vi "Get Table Object.vi"(8 "error in (no error)":errorcluster, 11 "Form Model in":refnum<class "Form Model.lvclass">) -> (0 "error out":errorcluster, 2 "Table":refnum<class "Basic Table.lvclass">, 3 "Form Model out":refnum<class "Form Model.lvclass">)   [LabVIEW 2020, in "Form Model.lvlib" / "Form Model.lvclass"]
uses:
  Form Model.lvclass
  Database OOP/Table Libraries/Basic Table/Basic Table Class/Basic Table.lvclass
  Form Model.lvclass/Form Model.ctl
  <vilib>/ActorFramework/Reply Msg/Reply Msg.lvclass/Reply Msg.ctl
  <vilib>/ActorFramework/Message Enqueuer/Message Enqueuer.lvclass/Message Enqueuer.ctl
  <vilib>/ActorFramework/Reply Msg/Send Message And Wait For Response.vi
  <vilib>/ActorFramework/Message Enqueuer/Enqueue.vi
  Panel Form Controller Messages/Get Table Msg/Get Table Msg.lvclass
  C:/Program Files (x86)/National Instruments/LabVIEW 2020/vi.lib/ActorFramework/Reply Msg/Reply Msg.lvclass
  <vilib>/ActorFramework/Reply Msg/Reply Msg.lvclass
  C:/Program Files (x86)/National Instruments/LabVIEW 2020/vi.lib/ActorFramework/Message/Message.lvclass
  <vilib>/ActorFramework/Message Priority Queue/Priority Enqueue.vi
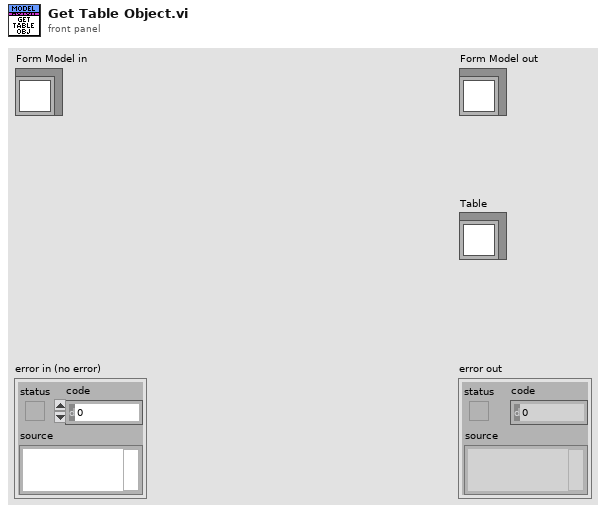
[diagram p1: front panel]
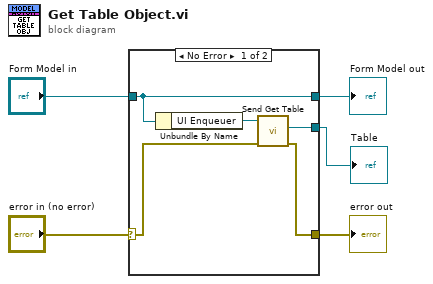
[diagram p0: block diagram]
diagram:
  n1 = case shown="No Error" "error in (no error)" {
    selector: "error in (no error)" -> [w7 w12]
    tunnel: [w6 w12] -> w4
    tunnel: "Form Model in" -> [w10 w11]
    tunnel: [w10 w11] -> w2
    tunnel: [w8 _] -> w1
    frame No Error {
      n2 = Unbundle By Name(w10) -> ("UI Enqueuer"=w9:refnum<class "Message Enqueuer.lvclass">)
      n3 = call "Send Get Table.vi"("error in (no error)"=w7, "Message Enqueuer"=w9) -> ("error out"=w6:errorcluster, "Table"=w8:refnum<class "Basic Table.lvclass">)  [unwired: 6 in, 2 out]
    }
    frame Error {
    }
  }
  "error out" <- w4
  "Form Model out" <- w2
  "Table" <- w1
